vi "Graphics test.vi"() -> ()   [LabVIEW 2013]
panel:
  out "2D Picture":picture
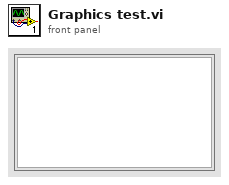
[diagram p1: front panel]
types:
  T1 = typedef "imagedata.ctl" = cluster{"image type":i32, "image depth":i32, "image":u8[], "mask":u8[], "colors":u32[], "Rectangle":cluster{"left":i16, "top":i16, "right":i16, "bottom":i16}}
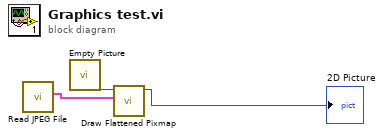
[diagram p0: block diagram]
diagram:
  n1 = call <vilib>:"Read JPEG File.vi"() -> ("image data"=w3:T1)  [unwired: 9 in, 2 out]
  n2 = call "Empty Picture"() -> ("empty picture"=w1:picture)
  n3 = call <vilib>:"Draw Flattened Pixmap.vi"("image data"=w3, "picture"=w1) -> ("new picture"=→"2D Picture":picture)  [unwired: 7 in]
